vi "HFRR ADV v011 new software.vi"() -> ()   [LabVIEW 2025] (continued)
              frame #3 {
                n3057 = disable-structure shown="Disabled" {
                  frame Disabled {
                    n3058 = local read "String 10"() -> (w3814:string)
                    n3059 = Concatenate Strings("C:\\LAB-IQ-NXT\\Data\\" ("string"), w3814, ".jpg" ("string")) -> (w3812:string)
                    n3060 = String To Path(string=w3812) -> (path=w3811:path)
                    n3061 = Delete(path (use dialog)=w3811) -> ()  [unwired: 4 in, 3 out]
                  }
                  frame Enabled {
                  }
                }
                n3062 = local write "Print 2"(FALSE ("Print")) -> ()
              }
            }
          }
        }
      }
    }
    n3063 = property on="SetTemp" class="DigNum (strict)"("Disabled"=w1752) -> ()  [unwired: 2 in, 2 out]
    n3064 = Multiply(x=w1742, y=w1744) -> (x*y=w1743:dbl)
    n3065 = local read "MWSD"() -> (w1741:dbl)
    n3066 = Add(x=w1743, y=w1741) -> (x+y=→"WS1.4":dbl)
    n3067 = Wait (ms)(milliseconds to wait=u32 50) -> ()  [unwired: 1 out]
    n3068 = Wait (ms)(milliseconds to wait=u32 50) -> ()  [unwired: 1 out]
    n3069 = local read "Quit"() -> (w1740:bool)
  }
  n3070 = VISA Close(VISA resource name=w52, error in (no error)=w51) -> (error out=w49:errorcluster)
  n3071 = call <vilib>:"Clear Errors.vi"("error in (no error)"=w49) -> ()  [unwired: 5 in, 2 out]
  n3072 = VISA Close(VISA resource name=w37, error in (no error)=w36) -> ()  [unwired: 1 out]
  n3073 = while {
    tunnel: [w3975] -> w46
    shift-right: [w3968] -> _
    shift-left: 0.0 -> [w3971]
    shift-right: [w3967] -> _
    shift-left: 0.0 -> [w3970]
    shift-right: [w3966] -> _
    shift-left: 400.0 ("vc_cmd") -> [w3969]
    stop <- w3975 stop-if-true
    # "PID LOGIC"
    n3074 = local read "RUN"() -> (w3973:bool)
    n3075 = local read "Auto Start Temp"() -> (w3962:bool)
    n3076 = local read "Auto Start Test"() -> (w3972:bool)
    n3077 = local read "START TEMP"() -> (w3964:bool)
    n3078 = And(x=w3962, y=w3972) -> (x .and. y?=w3963:bool)
    n3079 = Or(x=w3973, y=w3963) -> (x .or. y?=w3974:bool)
    n3080 = And(x=w3974, y=w3964) -> (x .and. y?=w3965:bool)
    n3081 = Wait (ms)(milliseconds to wait=u32 20) -> ()  [unwired: 1 out]
    n3082 = case shown="True" w3965 {
      tunnel: [400.0 ("out_vc_cmd") w3995] -> w3966
      tunnel: [w3978 w3997] -> w3967
      tunnel: [w3978 w3996] -> w3968
      tunnel: w3971 -> [_ w3986]
      tunnel: w3970 -> [_ w3985]
      tunnel: w3969 -> [_ w3984]
      frame False {
        w3978 = 0.0 ("error_out")
      }
      frame True {
        n3083 = local read "Set Strk"() -> (w3981:dbl)
        n3084 = local read "LVDT STROKE"() -> (w3979:dbl)
        n3085 = Add(x=w3981, y="Add up Stroke") -> (x+y=w3982:dbl)
        n3086 = formula code="// Zero-Hardcode Explicit Positional-Form PID Engine\n// Inputs: target_stroke, measured_stroke, dt, prev_error, integral_accumulator_in, prev_vc_cmd\n//         kp, ki, kd, max_step_change, max_amplitude, min_amplitude, startup_cmd\n// Outputs: vc_cmd, error_out, out_error, integral_accumulator_out, out_vc_cmd\n\n// 1. Calculate Tracking Error\nfloat current_error = target_stroke - measured_stroke;\nerror_out = current_error;\n\n// 2. Compute Proportional Term\nfloat p_term = kp * current_error;\n\n// 3. Compute Derivative Term\nfloat d_term = 0.0;\nif (dt > 0.0) {\n    d_term = kd * ((current_error - prev_error) / dt);\n}\n\n// 4. Update and Accumulate Integral Term\nfloat current_integral = integral_accumulator_in + (current_error * dt);\nfloat i_term = ki * current_integral;\n\n// 5. Calculate Ideal Target Command\nfloat ideal_command = startup_cmd + p_term + i_term + d_term;\n\n// 6. Anti-Windup Protection (Back-calculation method)\nif (ideal_command > max_amplitude) {\n    float excess = ideal_command - max_amplitude;\n    if (ki > 0.0) {\n        current_integral -= excess / ki;\n    }\n    ideal_command = max_amplitude;\n} else if (ideal_command < min_amplitude) {\n    float excess = ideal_command - min_amplitude;\n    if (ki > 0.0) {\n        current_integral -= excess / ki;\n    }\n    ideal_command = min_amplitude;\n}\n\n// 7. Apply Loop Rate Limiting (Protects voice coil from large voltage steps)\nfloat raw_adjustment = ideal_command - prev_vc_cmd;\n\nif (raw_adjustment > max_step_change) {\n    raw_adjustment = max_step_change;\n} else if (raw_adjustment < -max_step_change) {\n    raw_adjustment = -max_step_change;\n}\n\nfloat next_vc_cmd = prev_vc_cmd + raw_adjustment;\n\n// Final Output Safety Safeguard Clamping\nif (next_vc_cmd > max_amplitude) {\n    next_vc_cmd = max_amplitude;\n} else if (next_vc_cmd < min_amplitude) {\n    next_vc_cmd = min_amplitude;\n}\n\n// 8. Map to Shift Registers for memory persistence\nvc_cmd = next_vc_cmd;\nout_error = current_error;                     \nintegral_accumulator_out = current_integral;  \nout_vc_cmd = next_vc_cmd;"("target_stroke"=w3982, "measured_stroke"=w3979, "dt"="dt", "integral_accumulator_in"=w3985, "prev_error"=w3986, "prev_vc_cmd"=w3984, "kp"="kp", "ki"="ki", "kd"="kd", "max_step_change"="max_step_change", "max_amplitude"="max_amplitude", "min_amplitude"="min_amplitude", "startup_cmd"="startup_cmd") -> ("vc_cmd"=w4001:dbl, "out_error"=w3996:dbl, "integral_accumulator_out"=w3997:dbl, "out_vc_cmd"=w3995:dbl)  [unwired: 1 out]
        "output Vpp" <- w4001
        n3087 = Number To Fractional String(number=w4001, precision (6)=i16 1) -> (F-format string=w3999:string)  [unwired: 2 in]
        n3088 = Concatenate Strings("DAC;" ("string"), w3999) -> (w3983:string)
        n3089 = local write "Command"(w3983) -> ()
        "prev_error" <- w3986
        "integral_accumulator_in" <- w3985
        "prev_vc_cmd" <- w3984
      }
    }
    n3090 = local read "Quit"() -> (w3975:bool)
  }
  n3091 = Or(x=w42, y=w41) -> (x .or. y?=w43:bool)
  n3092 = Or(x=w39, y=w43) -> (x .or. y?=w48:bool)
  n3093 = control-ref of="new picture"() -> ()  [unwired: 1 out]
  n3094 = Or(x=w54, y=w48) -> (x .or. y?=w45:bool)
  n3095 = Or(x=w45, y=w46) -> (x .or. y?=w40:bool)
  n3096 = while {
    tunnel: [w4002] -> w53
    i -> [w4009]
    stop <- w4002 stop-if-true
    n3097 = local read "Quit"() -> (w4002:bool)
    n3098 = Equal To 0?(x=w4009) -> (x = 0?=w4007:bool)
    n3099 = call "Elapsed Time3"("Time Target (s)"=45.0, "Auto Reset"=TRUE) -> ("Time has Elapsed"=w4006:bool)  [unwired: 10 in, 7 out]
    n3100 = Wait (ms)(milliseconds to wait=u32 50) -> ()  [unwired: 1 out]
    n3101 = Or(x=w4006, y=w4007) -> (x .or. y?=w4008:bool)
    n3102 = case shown="True" w4008 {
      frame False {
      }
      frame True {
        n3103 = call <vilib>:"System Exec.vi"("run minimized? (F)"=TRUE, "error in (no error)"="error in (no error)", "command line"="powercfg.exe -change -monitor-timeout-ac 0") -> ("error out"=w4020:errorcluster)  [unwired: 5 in, 3 out]
        n3104 = call <vilib>:"System Exec.vi"("run minimized? (F)"=TRUE, "error in (no error)"=w4020, "command line"="powercfg.exe -change -disk-timeout-ac 0") -> ("error out"=w4019:errorcluster)  [unwired: 5 in, 3 out]
        n3105 = call <vilib>:"System Exec.vi"("run minimized? (F)"=TRUE, "error in (no error)"=w4019, "command line"="powercfg.exe -change -standby-timeout-ac 0") -> ("error out"=w4018:errorcluster)  [unwired: 5 in, 3 out]
        n3106 = call <vilib>:"System Exec.vi"("run minimized? (F)"=TRUE, "error in (no error)"=w4018, "command line"="powercfg.exe -change -hibernate-timeout-ac 0") -> ("error out"=w4017:errorcluster)  [unwired: 5 in, 3 out]
        n3107 = call <vilib>:"Simple Error Handler.vi"("error in (no error)"=w4017) -> ("error out"=w4023:errorcluster)  [unwired: 4 in, 4 out]
        n3108 = call <vilib>:"Clear Errors.vi"("error in (no error)"=w4023) -> ("error out"=→"error out":errorcluster)  [unwired: 5 in, 1 out]
      }
    }
  }
  n3109 = Compound Arithmetic op=OR(w56, w40, w53) -> (w55:bool)
  n3110 = flat-sequence {
    tunnel: w55 -> [_]
    tunnel: [w4025] -> w18
    tunnel: w18 -> [_]
    frame #0 {
      n3111 = call "CLOSE CONNECTION.vi"() -> ("error out"=w4025:errorcluster)  [unwired: 11 in]
    }
    frame #1 {
      n3112 = Quit LabVIEW(quit? (T)=TRUE) -> ()
      n3113 = local write "Quit"(FALSE ("EXIT")) -> ()
    }
  }
  n3114 = property on="Heater Button" class="Bool (strict)"("Visible"=TRUE) -> ()  [unwired: 2 in, 2 out]
  n3115 = disable-structure shown="Disabled" {
    disable-tunnel: _ -> [w4031 _]
    disable-tunnel: _ -> [w4028 _]
    disable-tunnel: _ -> [w4029 _]
    frame Disabled {
      n3116 = disable-structure shown="Disabled" {
        disable-tunnel: [w4038 _] -> w4030
        frame Disabled {
          n3117 = while {
            shift-right: [w4080] -> w4036
            shift-left: errorcluster {"status"=TRUE, "code"=0, "source"="Init"} ("error out") -> [w4045]
            shift-right: [w4079] -> w4035
            shift-left: _ -> [w4046]
            shift-right: [w4078] -> _
            shift-left: "" -> [w4077]
            tunnel: [w4039] -> w4038
            shift-right: ["Set Rh"] -> _
            shift-left: 0.0 ("Set Rh") -> [w4071]
            tunnel: [w4048] -> _
            i -> [w4048]
            stop <- w4039 stop-if-true
            n3118 = flat-sequence {
              tunnel: w4045 -> [w4083]
              tunnel: [w4083] -> w4044
              frame #0 {
                n3119 = Wait (ms)(milliseconds to wait=u32 200) -> ()  [unwired: 1 out]
              }
            }
            n3120 = local read "Com Port 3"() -> (w4047:refnum<visa-resource-name>)
            n3121 = local read "Humidity Str Rec"() -> (w4049:string)
            n3122 = Not Equal?(x="Set Rh", y=w4071) -> (x != y?=w4076:bool)
            n3123 = Number To Decimal String(number="Set Rh") -> (decimal integer string=w4074:string)  [unwired: 1 in]
            n3124 = Not Equal?(x=w4047, y=w4046) -> (x != y?=w4042:bool)
            n3125 = Concatenate Strings("#setPoint00" ("string"), w4074) -> (w4075:string)
            n3126 = case shown="False" w4076 {
              tunnel: w4075 -> [_ w4095]
              frame False {
                n3127 = local read "Humidity"() -> (w4092:bool)
                n3128 = case shown="True" w4092 {
                  frame False {
                    n3129 = local write "Humidity Str Send"("stop" ("Humidity Str Send")) -> ()
                  }
                  frame True {
                    n3130 = local write "Humidity Str Send"("start" ("Humidity Str Send")) -> ()
                  }
                }
              }
              frame True {
                n3131 = local write "Humidity Str Send"(w4095) -> ()
              }
            }
            n3132 = Or(x=w4042) -> (y=w4040:bool, x .or. y?=w4041:bool)
            n3133 = String Subset(string=w4049, offset (0)=7) -> (substring=w4064:string)  [unwired: 1 in]
            n3134 = Match Pattern(string=w4049, regular expression="?") -> (offset past match=w4067:i32)  [unwired: 1 in, 3 out]
            n3135 = Match Pattern(string=w4049, regular expression="v") -> (offset past match=w4070:i32)  [unwired: 1 in, 3 out]
            n3136 = case shown="True" w4041 {
              tunnel: w4044 -> [w4081 _]
              tunnel: [w4081 errorcluster {"status"=TRUE, "code"=0, "source"="Init"} ("error out")] -> w4043
              frame False {
              }
              frame True {
              }
            }
            n3137 = Equal?(x=w4067, y=-1) -> (x = y?=w4051:bool)
            n3138 = Match Pattern(string=w4064, regular expression="g") -> (after substring=w4065:string, offset past match=w4056:i32)  [unwired: 1 in, 2 out]
            n3139 = Match Pattern(string=w4064, regular expression="y") -> (after substring=w4063:string, offset past match=w4057:i32)  [unwired: 1 in, 2 out]
            n3140 = Greater?(x=w4057, y=w4056) -> (0:w4062:bool)
            n3141 = Greater Or Equal To 0?(x=w4057) -> (x >= 0?=w4054:bool)
            n3142 = Greater Or Equal To 0?(x=w4056) -> (x >= 0?=w4055:bool)
            n3143 = Or(x=w4054, y=w4055) -> (x .or. y?=w4053:bool)
            n3144 = Greater Or Equal To 0?(x=w4070) -> (x >= 0?=w4052:bool)
            n3145 = Select(t=w4063, s=w4062, f=w4065) -> (s? t:f=w4058:string)
            n3146 = case shown="Error" w4043 {
              selector: w4043 -> [w4108 w4154]
              tunnel: [w4106 w4147] -> w4080
              tunnel: w4046 -> [w4109 w4153]
              tunnel: [w4107 w4156] -> w4079
              tunnel: w4077 -> [w4096 w4155]
              tunnel: [w4103 w4155] -> w4078
              frame No Error {
                n3147 = call "Elapsed Time7"() -> ("Time has Elapsed"=w4102:bool)  [unwired: 12 in, 7 out]
                n3148 = Not Equal?(x="Humidity Str Send", y=w4096) -> (x != y?=w4098:bool)
                n3149 = Or(x=w4098, y=w4102) -> (x .or. y?=w4101:bool)
                n3150 = Select(t="Humidity Str Send", s=w4098, f="vals" ("regular expression")) -> (s? t:f=w4097:string)
                n3151 = Or(x=w4101, y="Send") -> (x .or. y?=w4105:bool)
                n3152 = case shown="True" w4105 {
                  tunnel: [w4112 w4117] -> w4106
                  tunnel: w4109 -> [w4111 w4125]
                  tunnel: w4108 -> [w4112 w4124]
                  tunnel: [w4111 w4118] -> w4107
                  tunnel: w4097 -> [_ w4123]
                  tunnel: [w4110 w4114] -> w4103
                  tunnel: "Humidity Str Send" -> [_ w4115]
                  tunnel: w4098 -> [_ w4116]
                  tunnel: w4096 -> [w4110 w4113]
                  frame False {
                  }
                  frame True {
                    n3153 = flat-sequence {
                      tunnel: w4125 -> [w4133]
                      tunnel: w4124 -> [w4132]
                      tunnel: w4123 -> [w4129]
                      tunnel: [w4131] -> w4122
                      tunnel: [w4130] -> w4121
                      tunnel: w4122 -> [w4136]
                      tunnel: w4121 -> [w4135]
                      tunnel: [w4136] -> w4120
                      tunnel: [w4135] -> w4119
                      tunnel: w4120 -> [w4143]
                      tunnel: w4119 -> [w4142]
                      tunnel: [w4141] -> w4118
                      tunnel: [w4140] -> w4117
                      frame #0 {
                        n3154 = local write "Ser Led"(TRUE ("Boolean 4")) -> ()
                        n3155 = Concatenate Strings(w4129, "\r") -> (w4128:string)
                        n3156 = VISA Write(VISA resource name=w4133, write buffer=w4128, error in (no error)=w4132) -> (VISA resource name out=w4131:refnum<visa-resource-name>, error out=w4130:errorcluster)  [unwired: 1 out]
                      }
                      frame #1 {
                        n3157 = Wait (ms)(milliseconds to wait="wait") -> ()  [unwired: 1 out]
                      }
                      frame #2 {
                        w4138 = FALSE ("Send")
                        n3158 = property class="Instr"(reference=w4143, error in=w4142) -> (reference out=w4144:refnum<visa-resource-name>, error out=w4145:errorcluster, "Serial Settings:Number of Bytes at Serial Port"=w4137:u32)
                        n3159 = local write "Send"(w4138) -> ()
                        n3160 = local write "Ser Led"(w4138) -> ()
                        n3161 = VISA Read(VISA resource name=w4144, byte count=w4137, error in (no error)=w4145) -> (VISA resource name out=w4141:refnum<visa-resource-name>, read buffer=→"Humidity Str Rec":string, error out=w4140:errorcluster)  [unwired: 1 out]
                      }
                    }
                    n3162 = Select(t=w4115, s=w4116, f=w4113) -> (s? t:f=w4114:string)
                  }
                }
              }
              frame Error {
                w4161 = u16 0 items=["None"=0, "XON/XOFF"=1, "RTS/CTS"=2, "DTR/DSR"=4] ("flow control")
                w4157 = u16 0 items=["None", "Odd", "Even", "Mark", "Space"] ("parity")
                w4160 = u16 10 items=["1.0"=10, "1.5"=15, "2.0"=20] ("stop bits")
                n3163 = VISA Close(VISA resource name=w4153, error in (no error)=w4154) -> (error out=w4152:errorcluster)
                n3164 = local write "humid"("" ("humid")) -> ()
                n3165 = local write "Humidity Str Rec"("" ("Humidity Str Rec")) -> ()
                n3166 = call <vilib>:"Clear Errors.vi"("error in (no error)"=w4152) -> ("error out"=w4151:errorcluster)  [unwired: 5 in, 1 out]
                n3167 = local read "Com Port 3"() -> (w4150:refnum<visa-resource-name>)
                n3168 = call-poly "VISA Configure Serial Port"("VISA resource name"=w4150, "timeout (10sec)"=u32 1000, "termination char\n(0xA = '\\n' = LF)"=u8 10 ("termination char\n(0xA = '\\n' = LF)"), "Enable Termination\nChar (T)"=FALSE ("Enable Termination Char (T)"), "data bits (8)"=u16 8 ("data bits"), "parity (0:none)"=w4157, "error in (no error)"=w4151, "stop bits (10: 1 bit)"=w4160, "flow control (0:none)"=w4161) -> ("VISA resource name out"=w4156:refnum<visa-resource-name>, "baud rate (9600)"=w4148:u32, "error out"=w4147:errorcluster)  [unwired: 4 in]
              }
            }
            n3169 = Compound Arithmetic op=AND(w4052, w4051, w4053) -> (w4050:bool)
            n3170 = case shown="True" w4050 {
              tunnel: w4049 -> [_ _]
              tunnel: w4058 -> [_ w4088]
              frame False {
              }
              frame True {
                w4086 = " " ("regular expression")
                n3171 = Match Pattern(string=w4088, regular expression=" ") -> (after substring=w4090:string)  [unwired: 1 in, 3 out]
                n3172 = Match Pattern(string=w4090, regular expression=w4086) -> (before substring=→"humid":string, after substring=w4087:string)  [unwired: 1 in, 2 out]
                n3173 = Match Pattern(string=w4087, regular expression=w4086) -> (before substring=→"temp_@Rh sensor":string)  [unwired: 1 in, 3 out]
              }
            }
            n3174 = local read "Quit"() -> (w4039:bool)
          }
          n3175 = VISA Close(VISA resource name=w4035, error in (no error)=w4036) -> (error out=w4032:errorcluster)
          n3176 = call <vilib>:"Clear Errors.vi"("error in (no error)"=w4032) -> ()  [unwired: 5 in, 2 out]
        }
        frame Enabled {
        }
      }
    }
    frame Enabled {
    }
  }
  n3177 = while {
    tunnel: [w4168] -> _
    i -> [w4168]
    stop <- w4164 stop-if-true
    # "Langauage selection"
    n3178 = Equal?(x="Lan flag", y=22.0) -> ()  [unwired: 1 out]
    n3179 = disable-structure shown="Disabled" {
      frame Disabled {
        n3180 = stacked-sequence {
          frame #0 {
            n3181 = case shown="\"Russian\"" "Language Selection" {
              tunnel: [0 1] -> w4170
              frame "English", Default {
              }
              frame "Russian" {
              }
            }
            n3182 = for {
              N: 130 -> [_]
              tunnel: "Table" -> [w4179]
              tunnel: w4170 -> [w4178]
              i -> [w4177]
              n3183 = Index Array(array=w4179, index (row)=w4177, index (col)=w4178) -> (element=w4176:string)
              n3184 = case shown="123" w4177 {
                tunnel: w4176 -> [w4180 w4181 _ w4182 w4183 w4184 w4185 w4186 w4187 w4188 w4189 w4190 w4191 w4192 w4193 w4194 w4195 w4196 w4197 w4198 w4199 w4200 w4201 w4202 w4203 w4204 w4205 w4206 w4207 _ _ w4208 w4209 w4210 w4211 w4212 w4213 w4222 w4229 w4236 w4243 w4247 w4250 w4253 w4255 w4257 w4258 w4259 w4260 w4261 w4262 w4263 w4264 w4265 w4266 w4267 w4268 w4269 w4270 w4271 w4272 w4273 w4274 w4275 w4276 w4277 w4278 w4279 w4280 w4281 w4282 w4283 w4284 w4285 w4286 w4287 w4288 w4289 w4290 w4291 w4292 w4293 w4294 w4295 w4296 w4297 w4298 w4299 w4300 w4301 w4302 w4303 w4304 w4305 w4306 w4307 w4308 w4309 w4310 w4311 w4312 w4313 w4314 w4315 w4316 _ w4317 w4318 w4319 w4320 w4321 w4322 w4323 w4324 w4325 w4326 w4327 w4328 w4329 _ w4330 w4331 w4332 w4333 w4334 w4335 _]
                frame 0 {
                  n3185 = local write "S"(w4180) -> ()
                }
                frame 1 {
                  n3186 = local write "S 2"(w4181) -> ()
                }
                frame 2 {
                }
                frame 3 {
                  n3187 = local write "S 4"(w4182) -> ()
                }
                frame 4 {
                  n3188 = property on="FILE" class="Str"("Caption.Text"=w4183) -> ()  [unwired: 2 in, 2 out]
                }
                frame 5 {
                  n3189 = property on="Fuel Discription :" class="Str"("Caption.Text"=w4184) -> ()  [unwired: 2 in, 2 out]
                }
                frame 6 {
                  n3190 = property on="Remarks :" class="Str"("Caption.Text"=w4185) -> ()  [unwired: 2 in, 2 out]
                }
                frame 7 {
                  n3191 = property on="Save & Continue" class="Bool (strict)"("Boolean Text.Text"=w4186) -> ()  [unwired: 2 in, 2 out]
                }
                frame 8 {
                }
                frame 9 {
                  n3192 = property on="Set Hz" class="DigNum (strict)"("Caption.Text"=w4188) -> ()  [unwired: 2 in, 2 out]
                }
                frame 10 {
                  "String 3" <- w4189
                }
                frame 11 {
                  n3193 = property on="NORMAL LOAD" class="DigNum (strict)"("Caption.Text"=w4190) -> ()  [unwired: 2 in, 2 out]
                }
                frame 12 {
                  "String 5" <- w4191
                }
                frame 13 {
                  n3194 = property on="Set Temp" class="DigNum (strict)"("Caption.Text"=w4192) -> ()  [unwired: 2 in, 2 out]
                }
                frame 14 {
                  n3195 = local write "S 15"(w4193) -> ()
                }
                frame 15 {
                  n3196 = property on="Set Rh" class="DigNum (strict)"("Caption.Text"=w4194) -> ()  [unwired: 2 in, 2 out]
                }
                frame 16 {
                  "String 13" <- w4195
                  "String 26" <- w4195
                }
                frame 17 {
                  n3197 = local write "S 18"(w4196) -> ()
                }
                frame 18 {
                  "String 17" <- w4197
                }
                frame 19 {
                  n3198 = property on="test time" class="DigNum (strict)"("Caption.Text"=w4198) -> ()  [unwired: 2 in, 2 out]
                }
                frame 20 {
                  "String 18" <- w4199
                  "String 22" <- w4199
                }
                frame 21 {
                  n3199 = property on="Elapsed time" class="DigNum (strict)"("Caption.Text"=w4200) -> ()  [unwired: 2 in, 2 out]
                }
                frame 22 {
                  n3200 = property on="Samplingtime 2" class="DigNum (strict)"("Caption.Text"=w4201) -> ()  [unwired: 2 in, 2 out]
                }
                frame 23 {
                  "String 21" <- w4202
                }
                frame 24 {
                  n3201 = property on="Countdown" class="DigNum (strict)"("Caption.Text"=w4203) -> ()  [unwired: 2 in, 2 out]
                }
                frame 25 {
                  n3202 = property on="Countdown 2" class="DigNum (strict)"("Caption.Text"=w4204) -> ()  [unwired: 2 in, 2 out]
                }
                frame 26 {
                  n3203 = property on="Engage" class="Bool (strict)"("Boolean Text.Text"=w4205) -> ()  [unwired: 2 in, 2 out]
                }
                frame 27 {
                  n3204 = property on="Boolean  4" class="Bool (strict)"("Boolean Text.Text"=w4206) -> ()  [unwired: 2 in, 2 out]
                }
                frame 28 {
                  n3205 = property on="Test \nStatus" class="Bool (strict)"("Boolean Text.Text"=w4207) -> ()  [unwired: 2 in, 2 out]
                }
                frame 29 {
                }
                frame 30 {
                }
                frame 31 {
                }
                frame 32 {
                  n3206 = property on="RSTCOF" class="Bool"("Boolean Text.Text"=w4209) -> ()  [unwired: 2 in, 2 out]
                  n3207 = property on="RST FF" class="Bool"("Boolean Text.Text"=w4209) -> ()  [unwired: 2 in, 2 out]
                  n3208 = property on="RST TEMP" class="Bool"("Boolean Text.Text"=w4209) -> ()  [unwired: 2 in, 2 out]
                  n3209 = property on="RSTV1 3" class="Bool"("Boolean Text.Text"=w4209) -> ()  [unwired: 2 in, 2 out]
                  n3210 = property on="rstv2" class="Bool"("Boolean Text.Text"=w4209) -> ()  [unwired: 2 in, 2 out]
                  n3211 = property on="RSTV1 2" class="Bool"("Boolean Text.Text"=w4209) -> ()  [unwired: 2 in, 2 out]
                  n3212 = property on="RST CP" class="Bool"("Boolean Text.Text"=w4209) -> ()  [unwired: 2 in, 2 out]
                }
                frame 33 {
                  "S 61" <- w4210
                }
                frame 34 {
                  "String 23" <- w4211
                }
                frame 35 {
                  n3213 = property on="Rh Before" class="DigNum (strict)"("Caption.Text"=w4212) -> ()  [unwired: 2 in, 2 out]
                }
                frame 36 {
                  n3214 = Match Pattern(string=w4213, regular expression=",") -> (before substring=→"bs":string, after substring=→"as":string)  [unwired: 1 in, 2 out]
                  n3215 = property on="Rh After" class="DigNum (strict)"("Caption.Text"=w4213) -> ()  [unwired: 2 in, 2 out]
                }
                frame 37 {
                  n3216 = Match Pattern(string=w4222, regular expression=",") -> (before substring=w4221:string, after substring=w4220:string)  [unwired: 1 in, 2 out]
                  "bs" <- w4221
                  "as" <- w4220
                  n3217 = Concatenate Strings(w4221, w4220) -> (w4217:string)
                  n3218 = property on="Humidity before test 2" class="DigNum (strict)"("Caption.Text"=w4217) -> ()  [unwired: 2 in, 2 out]
                  n3219 = property on="Humidity before test" class="DigNum (strict)"("Caption.Text"=w4217) -> ()  [unwired: 2 in, 2 out]
                  n3220 = Concatenate Strings(w4217, "=" ("string")) -> (w4218:string)
                  n3221 = local write "S 38"(w4218) -> ()
                }
                frame 38 {
                  n3222 = Match Pattern(string=w4229, regular expression=",") -> (before substring=w4228:string, after substring=w4227:string)  [unwired: 1 in, 2 out]
                  "bs" <- w4228
                  "as" <- w4227
                  n3223 = Concatenate Strings(w4228, w4227) -> (w4224:string)
                  n3224 = property on="Humidity after test 2" class="DigNum (strict)"("Caption.Text"=w4224) -> ()  [unwired: 2 in, 2 out]
                  n3225 = Concatenate Strings(w4224, "=" ("string")) -> (w4226:string)
                  n3226 = property on="Humidity after test" class="DigNum (strict)"("Caption.Text"=w4224) -> ()  [unwired: 2 in, 2 out]
                  n3227 = local write "S 39"(w4226) -> ()
                }
                frame 39 {
                  n3228 = Match Pattern(string=w4236, regular expression=",") -> (before substring=w4235:string, after substring=w4234:string)  [unwired: 1 in, 2 out]
                  "bs" <- w4235
                  "as" <- w4234
                  n3229 = Concatenate Strings(w4235, w4234) -> (w4231:string)
                  n3230 = property on="Temperature before test 2" class="DigNum (strict)"("Caption.Text"=w4231) -> ()  [unwired: 2 in, 2 out]
                  n3231 = property on="Temperature before test" class="DigNum (strict)"("Caption.Text"=w4231) -> ()  [unwired: 2 in, 2 out]
                  n3232 = Concatenate Strings(w4231, "=" ("string")) -> (→"String 34":string)
                }
                frame 40 {
                  n3233 = Match Pattern(string=w4243, regular expression=",") -> (before substring=w4242:string, after substring=w4241:string)  [unwired: 1 in, 2 out]
                  "bs" <- w4242
                  "as" <- w4241
                  n3234 = Concatenate Strings(w4242, w4241) -> (w4238:string)
                  n3235 = property on="Temperature after test 2" class="DigNum (strict)"("Caption.Text"=w4238) -> ()  [unwired: 2 in, 2 out]
                  n3236 = Concatenate Strings(w4238, "=" ("string")) -> (→"String 35":string)
                  n3237 = property on="Temperature after test" class="DigNum (strict)"("Caption.Text"=w4238) -> ()  [unwired: 2 in, 2 out]
                }
                frame 41 {
                  n3238 = property on="AVP" class="DigNum (strict)"("Caption.Text"=w4247) -> ()  [unwired: 2 in, 2 out]
                  n3239 = property on="AVP 2" class="DigNum (strict)"("Caption.Text"=w4247) -> ()  [unwired: 2 in, 2 out]
                  n3240 = Concatenate Strings(w4247, "=" ("string")) -> (→"String 36":string)
                }
                frame 42 {
                  n3241 = property on="MWSD" class="DigNum (strict)"("Caption.Text"=w4250) -> ()  [unwired: 2 in, 2 out]
                  n3242 = property on="MWSD 2" class="DigNum (strict)"("Caption.Text"=w4250) -> ()  [unwired: 2 in, 2 out]
                  n3243 = Concatenate Strings(w4250, "=" ("string")) -> (→"String 37":string)
                }
                frame 43 {
                  n3244 = property on="HCF 2" class="DigNum (strict)"("Caption.Text"=w4253) -> ()  [unwired: 2 in, 2 out]
                  n3245 = property on="HCF" class="DigNum (strict)"("Caption.Text"=w4253) -> ()  [unwired: 2 in, 2 out]
                  n3246 = Concatenate Strings(w4253, "=" ("string")) -> (→"String 38":string)
                }
                frame 44 {
                  n3247 = Concatenate Strings(w4255, "=" ("string")) -> (→"String 39":string)
                  n3248 = property on="WS1.4 2" class="DigNum (strict)"("Caption.Text"=w4255) -> ()  [unwired: 2 in, 2 out]
                  n3249 = property on="WS1.4" class="DigNum (strict)"("Caption.Text"=w4255) -> ()  [unwired: 2 in, 2 out]
                }
                frame 45 {
                  n3250 = property on="Save Results" class="Bool (strict)"("Boolean Text.Text"=w4257) -> ()  [unwired: 2 in, 2 out]
                }
                frame 46 {
                  n3251 = local write "S 47"(w4258) -> ()
                }
                frame 47 {
                  n3252 = local write "S 48"(w4259) -> ()
                }
                frame 48 {
                  n3253 = local write "S 49"(w4260) -> ()
                }
                frame 49 {
                  n3254 = local write "S 50"(w4261) -> ()
                }
                frame 50 {
                  n3255 = local write "S 51"(w4262) -> ()
                }
                frame 51 {
                  n3256 = local write "S 52"(w4263) -> ()
                }
                frame 52 {
                  n3257 = local write "S 53"(w4264) -> ()
                }
                frame 53 {
                  n3258 = local write "S 54"(w4265) -> ()
                }
                frame 54 {
                  n3259 = local write "S 55"(w4266) -> ()
                }
                frame 55 {
                  n3260 = local write "S 56"(w4267) -> ()
                }
                frame 56 {
                  n3261 = local write "S 57"(w4268) -> ()
                }
                frame 57 {
                  n3262 = local write "S 58"(w4269) -> ()
                }
                frame 58 {
                  n3263 = local write "S 59"(w4270) -> ()
                }
                frame 59 {
                  n3264 = local write "S 60"(w4271) -> ()
                }
                frame 60 {
                  n3265 = local write "S 62"(w4272) -> ()
                }
                frame 61 {
                  n3266 = local write "S 63"(w4273) -> ()
                }
                frame 62 {
                  n3267 = local write "S 64"(w4274) -> ()
                }
                frame 63 {
                  n3268 = local write "S 65"(w4275) -> ()
                }
                frame 64 {
                  n3269 = local write "S 66"(w4276) -> ()
                }
                frame 65 {
                  n3270 = local write "S 67"(w4277) -> ()
                }
                frame 66 {
                  n3271 = local write "S 68"(w4278) -> ()
                }
                frame 67 {
                  n3272 = local write "S 69"(w4279) -> ()
                }
                frame 68 {
                  n3273 = local write "S 70"(w4280) -> ()
                }
                frame 69 {
                  n3274 = local write "S 71"(w4281) -> ()
                }
                frame 70 {
                  n3275 = local write "S 72"(w4282) -> ()
                }
                frame 71 {
                  n3276 = local write "S 73"(w4283) -> ()
                }
                frame 72 {
                  n3277 = local write "S 74"(w4284) -> ()
                }
                frame 73 {
                  n3278 = local write "S 75"(w4285) -> ()
                }
                frame 74 {
                  n3279 = local write "S 76"(w4286) -> ()
                }
                frame 75 {
                  n3280 = local write "S 77"(w4287) -> ()
                }
                frame 76 {
                  n3281 = local write "S 78"(w4288) -> ()
                }
                frame 77 {
                  n3282 = local write "S 79"(w4289) -> ()
                }
                frame 79 {
                  n3283 = property on="Sample Temperature ( °C )" class="XYGraph (strict)"("Y Scale.Name Label.Text"=w4290) -> ()  [unwired: 2 in, 2 out]
                }
                frame 80 {
                  n3284 = local write "S 81"(w4291) -> ()
                  n3285 = property on="Humidity ( %RH )" class="XYGraph (strict)"("Y Scale.Name Label.Text"=w4291) -> ()  [unwired: 2 in, 2 out]
                }
                frame 78 {
                  n3286 = property on="Air Temperature  ( °C )" class="XYGraph (strict)"("X Scale.Name Label.Text"=w4292) -> ()  [unwired: 2 in, 2 out]
                  n3287 = property on="Humidity ( %RH )" class="XYGraph (strict)"("X Scale.Name Label.Text"=w4292) -> ()  [unwired: 2 in, 2 out]
                  n3288 = property on="Sample Temperature ( °C )" class="XYGraph (strict)"("X Scale.Name Label.Text"=w4292) -> ()  [unwired: 2 in, 2 out]
                  n3289 = property on="Coefficient Of Friction" class="XYGraph (strict)"("X Scale.Name Label.Text"=w4292) -> ()  [unwired: 2 in, 2 out]
                }
                frame 81 {
                  n3290 = property on="Air Temperature  ( °C )" class="XYGraph (strict)"("Y Scale.Name Label.Text"=w4293) -> ()  [unwired: 2 in, 2 out]
                }
                frame 82 {
                  n3291 = local write "S 84"(w4294) -> ()
                }
                frame 83 {
                  n3292 = local write "S 85"(w4295) -> ()
                }
                frame 84 {
                  n3293 = local write "S 86"(w4296) -> ()
                }
                frame 85 {
                  n3294 = local write "S 87"(w4297) -> ()
                }
                frame 86 {
                  n3295 = local write "S 88"(w4298) -> ()
                }
                frame 87 {
                }
                frame 88 {
                  n3296 = local write "S 90"(w4300) -> ()
                }
                frame 89 {
                  n3297 = local write "S 91"(w4301) -> ()
                }
                frame 90 {
                  n3298 = local write "S 92"(w4302) -> ()
                }
                frame 91 {
                  n3299 = local write "S 93"(w4303) -> ()
                }
                frame 92 {
                  n3300 = local write "S 94"(w4304) -> ()
                }
                frame 93 {
                  n3301 = local write "S 95"(w4305) -> ()
                }
                frame 94 {
                  n3302 = local write "S 96"(w4306) -> ()
                }
                frame 95 {
                  n3303 = local write "S 97"(w4307) -> ()
                }
                frame 96 {
                  n3304 = local write "S 98"(w4308) -> ()
                }
                frame 97 {
                  n3305 = local write "S 99"(w4309) -> ()
                }
                frame 98 {
                  n3306 = local write "S 100"(w4310) -> ()
                }
                frame 99 {
                  n3307 = local write "S 101"(w4311) -> ()
                }
                frame 100 {
                  n3308 = local write "S 102"(w4312) -> ()
                }
                frame 101 {
                  n3309 = local write "S 103"(w4313) -> ()
                }
                frame 102 {
                  n3310 = local write "S 104"(w4314) -> ()
                }
                frame 103 {
                  n3311 = local write "S 105"(w4315) -> ()
                }
                frame 104 {
                  n3312 = local write "S 106"(w4316) -> ()
                }
                frame 105 {
                }
                frame 106 {
                  n3313 = property on="OK Button 17" class="Bool (strict)"("Boolean Text.Text"=w4317) -> ()  [unwired: 2 in, 2 out]
                }
                frame 107 {
                  n3314 = property on="OK Button 16" class="Bool (strict)"("Boolean Text.Text"=w4318) -> ()  [unwired: 2 in, 2 out]
                }
                frame 108 {
                  n3315 = property on="TITTLE" class="Str"("Caption.Text"=w4319) -> ()  [unwired: 2 in, 2 out]
                }
                frame 109 {
                  "String 30" <- w4320
                }
                frame 110 {
                  n3316 = property on="Test Date" class="Str"("Caption.Text"=w4321) -> ()  [unwired: 2 in, 2 out]
                  "String 31" <- w4321
                }
                frame 111 {
                  n3317 = property on="Sample ID" class="Str"("Caption.Text"=w4322) -> ()  [unwired: 2 in, 2 out]
                  "String 32" <- w4322
                }
                frame 112 {
                  n3318 = property on="Tested by" class="Str"("Caption.Text"=w4323) -> ()  [unwired: 2 in, 2 out]
                  "String 33" <- w4323
                }
                frame 113 {
                  n3319 = property on="System Configured Printers 2" class="Arr (strict)"("Caption.Text"=w4324) -> ()  [unwired: 2 in, 2 out]
                }
                frame 114 {
                  n3320 = property on="Selected Printer" class="Str"("Caption.Text"=w4325) -> ()  [unwired: 2 in, 2 out]
                }
                frame 115 {
                  n3321 = property on="Select Printer 3" class="DigNum (strict)"("Caption.Text"=w4326) -> ()  [unwired: 2 in, 2 out]
                }
                frame 116 {
                  n3322 = property on="Print" class="Bool (strict)"("Boolean Text.Text"=w4327) -> ()  [unwired: 2 in, 2 out]
                }
                frame 117 {
                  "String 41" <- w4328
                }
                frame 118 {
                  n3323 = property on="tested by" class="Str"("Caption.Text"=w4329) -> ()  [unwired: 2 in, 2 out]
                }
                frame 119 {
                }
                frame 120 {
                  n3324 = property on="Export" class="Bool (strict)"("Boolean Text.Text"=w4330) -> ()  [unwired: 2 in, 2 out]
                }
                frame 121 {
                  n3325 = property on="TEMP INTERCEPT:" class="DigNum (strict)"("Caption.Text"=w4331) -> ()  [unwired: 2 in, 2 out]
                }
                frame 122 {
                  n3326 = property on="AIR TEMP INTERCEPT:" class="DigNum (strict)"("Caption.Text"=w4332) -> ()  [unwired: 2 in, 2 out]
                }
                frame 123 {
                  n3327 = property on="Select File Type" class="Enum (strict)"("Caption.Text"=w4333) -> ()  [unwired: 2 in, 2 out]
                }
                frame 124 {
                  n3328 = property on="s.NO" class="Str"("Caption.Text"=w4334) -> ()  [unwired: 2 in, 2 out]
                  "String 45" <- w4334
                }
                frame 125 {
                  n3329 = property on="trip1 8" class="Bool (strict)"("Boolean Text.Text"=w4335) -> ()  [unwired: 2 in, 2 out]
                }
                frame 126, Default {
                }
              }
            }
          }
          frame #1 {
            w4343 = TRUE ("Visible")
            n3330 = local read "S 91"() -> (w4360:string)
            n3331 = local read "S 90"() -> (w4359:string)
            n3332 = local read "S 88"() -> (w4358:string)
            n3333 = property on="File Path" class="Path"("Caption.Text"=w4359) -> ()  [unwired: 2 in, 2 out]
            n3334 = property on="SrvM CP" class="Bool (strict)"("Boolean Text.Text"=w4358) -> ()  [unwired: 2 in, 2 out]
            n3335 = local read "S 71"() -> (w4353:string)
            n3336 = local read "S 86"() -> (w4355:string)
            n3337 = local read "S 85"() -> (w4356:string)
            n3338 = local read "S 87"() -> (w4354:string)
            n3339 = local read "S 84"() -> (w4357:string)
            n3340 = local read "S 103"() -> (w4342:string)
            n3341 = local read "S 104"() -> (w4341:string)
            n3342 = property on="ENTER THE NEW PASSWORD" class="Str"("Caption.Text"=w4354) -> ()  [unwired: 2 in, 2 out]
            n3343 = property on="Password" class="Str"("Caption.Text"=w4356) -> ()  [unwired: 2 in, 2 out]
            n3344 = property on="ENTER CURRENT PASSWORD" class="Str"("Caption.Text"=w4355) -> ()  [unwired: 2 in, 2 out]
            n3345 = property on="EDIT" class="Bool (strict)"("Boolean Text.Text"=w4353) -> ()  [unwired: 2 in, 2 out]
            n3346 = property on="SAVE" class="Bool (strict)"("Boolean Text.Text"=w4357) -> ()  [unwired: 2 in, 2 out]
            n3347 = Build Array(w4342, w4341) -> (w4340:string[])
            n3348 = property on="Heater Button" class="Bool (strict)"("Strings [4]"=w4340) -> ()  [unwired: 2 in, 2 out]
            n3349 = property on="CH-HUMIDITY WET" class="DigNum (strict)"("Caption.Size to Text?"=w4343) -> ()  [unwired: 2 in, 2 out]
            n3350 = property on="CH-HUMIDITY DRY" class="DigNum (strict)"("Caption.Size to Text?"=w4343) -> ()  [unwired: 2 in, 2 out]
            n3351 = property on="CH-POWER -" class="DigNum (strict)"("Caption.Size to Text?"=w4343) -> ()  [unwired: 2 in, 2 out]
            n3352 = property on="CH-HEATER" class="DigNum (strict)"("Caption.Size to Text?"=w4343) -> ()  [unwired: 2 in, 2 out]
            n3353 = property on="CH-POWER +" class="DigNum (strict)"("Caption.Size to Text?"=w4343) -> ()  [unwired: 2 in, 2 out]
            n3354 = local read "S 92"() -> (w4352:string)
            n3355 = local read "S 93"() -> (w4351:string)
            n3356 = local read "S 105"() -> (w4338:string)
            n3357 = local read "S 106"() -> (w4337:string)
            n3358 = Build Array(w4352, w4351) -> ()  [unwired: 1 out]
            n3359 = Build Array(w4338, w4337) -> (w4339:string[])
            n3360 = local read "S 95"() -> (w4349:string)
            n3361 = local read "S 94"() -> (w4350:string)
            n3362 = local read "bs"() -> (w4365:string)
            n3363 = local read "as"() -> (w4366:string)
            n3364 = property on="Humidity" class="Bool (strict)"("Strings [4]"=w4339) -> ()  [unwired: 2 in, 2 out]
            n3365 = Concatenate Strings(w4365, "\r", w4366) -> ()  [unwired: 1 out]
            n3366 = property on="STROKE GAIN :" class="DigNum (strict)"("Caption.Text"=w4349) -> ()  [unwired: 2 in, 2 out]
            n3367 = property on="DISPLACEMENT :" class="DigNum (strict)"("Caption.Text"=w4350) -> ()  [unwired: 2 in, 2 out]
            n3368 = property on="Rh After" class="DigNum (strict)"("Caption.Size to Text?"=TRUE ("Caption.Size to Text")) -> ()  [unwired: 2 in, 2 out]
            n3369 = local read "S 48"() -> (w4389:string)
            n3370 = local read "S 50"() -> (w4387:string)
            n3371 = local read "S 51"() -> (w4386:string)
            n3372 = local read "S 49"() -> (w4388:string)
            n3373 = local read "S 52"() -> (w4385:string)
            n3374 = local read "as"() -> (w4370:string)
            n3375 = local read "bs"() -> (w4371:string)
            n3376 = local read "S 56"() -> (w4384:string)
            n3377 = local read "S 57"() -> (w4383:string)
            n3378 = local read "S 58"() -> (w4382:string)
            n3379 = local read "S 59"() -> (w4381:string)
            n3380 = property on="OPEN" class="Bool (strict)"("Boolean Text.Text"=w4385) -> ()  [unwired: 2 in, 2 out]
            n3381 = property on="OPEN 1" class="Bool (strict)"("Boolean Text.Text"=w4389) -> ()  [unwired: 2 in, 2 out]
            n3382 = property on="OPEN 2" class="Bool (strict)"("Boolean Text.Text"=w4388) -> ()  [unwired: 2 in, 2 out]
            n3383 = property on="OPEN 3" class="Bool (strict)"("Boolean Text.Text"=w4387) -> ()  [unwired: 2 in, 2 out]
            n3384 = property on="OPEN 4" class="Bool (strict)"("Boolean Text.Text"=w4386) -> ()  [unwired: 2 in, 2 out]
            n3385 = Concatenate Strings(w4371, "\r", w4370) -> ()  [unwired: 1 out]
            n3386 = local read "S 102"() -> (w4344:string)
            n3387 = property on="КОФ1" class="DigNum (strict)"("Caption.Text"=w4384) -> ()  [unwired: 2 in, 2 out]
            n3388 = local read "S 98"() -> (w4348:string)
            n3389 = local read "S 99"() -> (w4347:string)
            n3390 = local read "S 100"() -> (w4346:string)
            n3391 = local read "S 101"() -> (w4345:string)
            n3392 = property on="КОФ2" class="DigNum (strict)"("Caption.Text"=w4383) -> ()  [unwired: 2 in, 2 out]
            n3393 = property on="КОФ3" class="DigNum (strict)"("Caption.Text"=w4382) -> ()  [unwired: 2 in, 2 out]
            n3394 = property on="КОФ4" class="DigNum (strict)"("Caption.Text"=w4381) -> ()  [unwired: 2 in, 2 out]
            n3395 = local read "bs"() -> (w4369:string)
            n3396 = local read "as"() -> (w4368:string)
            n3397 = property on="CH-POWER +" class="DigNum (strict)"("Caption.Text"=w4348) -> ()  [unwired: 2 in, 2 out]
            n3398 = property on="CH-POWER -" class="DigNum (strict)"("Caption.Text"=w4347) -> ()  [unwired: 2 in, 2 out]
            n3399 = property on="CH-HEATER" class="DigNum (strict)"("Caption.Text"=w4346) -> ()  [unwired: 2 in, 2 out]
            n3400 = property on="CH-HUMIDITY DRY" class="DigNum (strict)"("Caption.Text"=w4345) -> ()  [unwired: 2 in, 2 out]
            n3401 = property on="CH-HUMIDITY WET" class="DigNum (strict)"("Caption.Text"=w4344) -> ()  [unwired: 2 in, 2 out]
            n3402 = local read "S 60"() -> (w4380:string)
            n3403 = local read "S 54"() -> (w4390:string)
            n3404 = Concatenate Strings(w4369, "\r", w4368) -> ()  [unwired: 1 out]
            n3405 = Concatenate Strings(w4390, w4380) -> ()  [unwired: 1 out]
            n3406 = local read "S 77"() -> (→"String 43":string)
            n3407 = local read "S 76"() -> (w4363:string)
            n3408 = local read "S 78"() -> (w4362:string)
            n3409 = local read "S 71"() -> (w4374:string)
            n3410 = local read "S 66"() -> (w4379:string)
            n3411 = local read "S 67"() -> (w4378:string)
            n3412 = local read "S 68"() -> (w4377:string)
            n3413 = local read "S 69"() -> (w4376:string)
            n3414 = local read "S 70"() -> (w4375:string)
            n3415 = property on="AIR TEMP" class="DigNum (strict)"("Caption.Text"=w4362) -> ()  [unwired: 2 in, 2 out]
            n3416 = property on="Set Strk" class="DigNum (strict)"("Caption.Text"=w4363) -> ()  [unwired: 2 in, 2 out]
            n3417 = property on="FRIC. FORCE :" class="DigNum (strict)"("Caption.Text"=w4379) -> ()  [unwired: 2 in, 2 out]
            n3418 = property on="TEMPERATURE :" class="DigNum (strict)"("Caption.Text"=w4378) -> ()  [unwired: 2 in, 2 out]
            n3419 = property on="SPEED OUT:" class="DigNum (strict)"("Caption.Text"=w4377) -> ()  [unwired: 2 in, 2 out]
            n3420 = property on="AIR TEMPERATURE :" class="DigNum (strict)"("Caption.Text"=w4376) -> ()  [unwired: 2 in, 2 out]
            n3421 = property on="HUMIDITY:" class="DigNum (strict)"("Caption.Text"=w4375) -> ()  [unwired: 2 in, 2 out]
            n3422 = property on="EDIT" class="Bool (strict)"("Boolean Text.Text"=w4374) -> ()  [unwired: 2 in, 2 out]
            n3423 = local read "S 79"() -> (w4361:string)
          }
          frame #2 {
          }
        }
        n3424 = local write "Lan flag"(10.0 ("Lan flag")) -> ()
      }
      frame Enabled {
      }
    }
    n3425 = Wait (ms)(milliseconds to wait=u32 2000) -> ()  [unwired: 1 out]
    n3426 = local read "Quit"() -> (w4164:bool)
  }
  n3427 = disable-structure shown="Disabled" {
    frame Disabled {
      n3428 = while {
        tunnel: [w4392] -> _
        i -> [w4392]
        stop <- w4391 continue-if-true
        n3429 = Wait (ms)(milliseconds to wait=u32 50) -> ()  [unwired: 1 out]
        n3430 = stacked-sequence {
          frame #0 {
            # "Controls Text color"
            # "Controls BG color"
            n3431 = property on="FILE" class="Str"("Text.Text Colors:Text Color"="SC  Text") -> ()  [unwired: 2 in, 2 out]
            n3432 = property on="Fuel Discription :" class="Str"("Text.Text Colors:Text Color"="SC  Text") -> ()  [unwired: 2 in, 2 out]
            n3433 = property on="tested by" class="Str"("Text.Text Colors:Text Color"="SC  Text") -> ()  [unwired: 2 in, 2 out]
            n3434 = property on="Remarks :" class="Str"("Text.Text Colors:Text Color"="SC  Text") -> ()  [unwired: 2 in, 2 out]
            n3435 = property class="DigNum (strict)"("Numeric Text.Text Colors:BG Color"="NC BG") -> ()  [unwired: 2 in, 2 out]
            n3436 = property class="DigNum (strict)"("Numeric Text.Text Colors:BG Color"="NC BG") -> ()  [unwired: 2 in, 2 out]
            n3437 = property class="DigNum (strict)"("Numeric Text.Text Colors:BG Color"="NC BG") -> ()  [unwired: 2 in, 2 out]
            n3438 = property class="DigNum (strict)"("Numeric Text.Text Colors:BG Color"="NC BG") -> ()  [unwired: 2 in, 2 out]
            n3439 = property class="DigNum (strict)"("Numeric Text.Text Colors:BG Color"="NC BG") -> ()  [unwired: 2 in, 2 out]
            n3440 = property class="DigNum (strict)"("Numeric Text.Text Colors:BG Color"="NC BG") -> ()  [unwired: 2 in, 2 out]
            n3441 = property class="DigNum (strict)"("Numeric Text.Text Colors:BG Color"="NC BG") -> ()  [unwired: 2 in, 2 out]
            n3442 = property class="DigNum (strict)"("Numeric Text.Text Colors:BG Color"="NC BG") -> ()  [unwired: 2 in, 2 out]
            n3443 = property class="DigNum (strict)"("Numeric Text.Text Colors:BG Color"="NC BG") -> ()  [unwired: 2 in, 2 out]
            n3444 = property class="DigNum (strict)"("Numeric Text.Text Colors:BG Color"="NC BG") -> ()  [unwired: 2 in, 2 out]
            n3445 = property class="DigNum (strict)"("Numeric Text.Text Colors:BG Color"="NC BG") -> ()  [unwired: 2 in, 2 out]
            n3446 = property class="DigNum (strict)"("Numeric Text.Text Colors:BG Color"="NC BG") -> ()  [unwired: 2 in, 2 out]
            n3447 = property on="FILE" class="Str"("Text.Text Colors:BG Color"="SC BG 3") -> ()  [unwired: 2 in, 2 out]
            n3448 = property on="Fuel Discription :" class="Str"("Text.Text Colors:BG Color"="SC BG 3") -> ()  [unwired: 2 in, 2 out]
            n3449 = property on="tested by" class="Str"("Text.Text Colors:BG Color"="SC BG 3") -> ()  [unwired: 2 in, 2 out]
            n3450 = property on="Remarks :" class="Str"("Text.Text Colors:BG Color"="SC BG 3") -> ()  [unwired: 2 in, 2 out]
            n3451 = property class="DigNum (strict)"("Numeric Text.Text Colors:Text Color"="NC Text") -> ()  [unwired: 2 in, 2 out]
            n3452 = property class="DigNum (strict)"("Numeric Text.Text Colors:Text Color"="NC Text") -> ()  [unwired: 2 in, 2 out]
            n3453 = property class="DigNum (strict)"("Numeric Text.Text Colors:Text Color"="NC Text") -> ()  [unwired: 2 in, 2 out]
            n3454 = property class="DigNum (strict)"("Numeric Text.Text Colors:Text Color"="NC Text") -> ()  [unwired: 2 in, 2 out]
            n3455 = property class="DigNum (strict)"("Numeric Text.Text Colors:Text Color"="NC Text") -> ()  [unwired: 2 in, 2 out]
            n3456 = property class="DigNum (strict)"("Numeric Text.Text Colors:Text Color"="NC Text") -> ()  [unwired: 2 in, 2 out]
            n3457 = property class="DigNum (strict)"("Numeric Text.Text Colors:Text Color"="NC Text") -> ()  [unwired: 2 in, 2 out]
            n3458 = property class="DigNum (strict)"("Numeric Text.Text Colors:Text Color"="NC Text") -> ()  [unwired: 2 in, 2 out]
            n3459 = property class="DigNum (strict)"("Numeric Text.Text Colors:Text Color"="NC Text") -> ()  [unwired: 2 in, 2 out]
            n3460 = property class="DigNum (strict)"("Numeric Text.Text Colors:Text Color"="NC Text") -> ()  [unwired: 2 in, 2 out]
            n3461 = property class="DigNum (strict)"("Numeric Text.Text Colors:Text Color"="NC Text") -> ()  [unwired: 2 in, 2 out]
            n3462 = property class="DigNum (strict)"("Numeric Text.Text Colors:Text Color"="NC Text") -> ()  [unwired: 2 in, 2 out]
            n3463 = property class="DigNum (strict)"("Numeric Text.Text Colors:Text Color"="NI Text  2") -> ()  [unwired: 2 in, 2 out]
            n3464 = property class="DigNum (strict)"("Numeric Text.Text Colors:Text Color"="NI Text  2") -> ()  [unwired: 2 in, 2 out]
            n3465 = property class="DigNum (strict)"("Numeric Text.Text Colors:Text Color"="NI Text  2") -> ()  [unwired: 2 in, 2 out]
            n3466 = property class="DigNum (strict)"("Numeric Text.Text Colors:Text Color"="NI Text  2") -> ()  [unwired: 2 in, 2 out]
            n3467 = property class="DigNum (strict)"("Numeric Text.Text Colors:Text Color"="NI Text  2") -> ()  [unwired: 2 in, 2 out]
            n3468 = property class="DigNum (strict)"("Numeric Text.Text Colors:Text Color"="NI Text  2") -> ()  [unwired: 2 in, 2 out]
            n3469 = property class="DigNum (strict)"("Numeric Text.Text Colors:Text Color"="NI Text  2") -> ()  [unwired: 2 in, 2 out]
            n3470 = property class="DigNum (strict)"("Numeric Text.Text Colors:Text Color"="NI Text  2") -> ()  [unwired: 2 in, 2 out]
            n3471 = property class="DigNum (strict)"("Numeric Text.Text Colors:Text Color"="NI Text  2") -> ()  [unwired: 2 in, 2 out]
            n3472 = property class="DigNum (strict)"("Numeric Text.Text Colors:Text Color"="NI Text  2") -> ()  [unwired: 2 in, 2 out]
            n3473 = property class="DigNum (strict)"("Numeric Text.Text Colors:Text Color"="NI Text  2") -> ()  [unwired: 2 in, 2 out]
            n3474 = property class="DigNum (strict)"("Numeric Text.Text Colors:Text Color"="NI Text  2") -> ()  [unwired: 2 in, 2 out]
            n3475 = property class="DigNum (strict)"("Numeric Text.Text Colors:Text Color"="NI Text  2") -> ()  [unwired: 2 in, 2 out]
            n3476 = property class="DigNum (strict)"("Numeric Text.Text Colors:Text Color"="NI Text  2") -> ()  [unwired: 2 in, 2 out]
            n3477 = property class="DigNum (strict)"("Numeric Text.Text Colors:Text Color"="NI Text  2") -> ()  [unwired: 2 in, 2 out]
            n3478 = property on="Coefficient Of Friction" class="XYGraph (strict)"("Plot Area:Colors:FG Color"="GFG  2", "Plot Area:Colors:BG Color"="GBG   2") -> ()  [unwired: 2 in, 2 out]
            n3479 = property on="Humidity ( %RH )" class="XYGraph (strict)"("Plot Area:Colors:FG Color"="GFG  2", "Plot Area:Colors:BG Color"="GBG   2") -> ()  [unwired: 2 in, 2 out]
            n3480 = property on="Air Temperature  ( °C )" class="XYGraph (strict)"("Plot Area:Colors:FG Color"="GFG  2", "Plot Area:Colors:BG Color"="GBG   2") -> ()  [unwired: 2 in, 2 out]
            n3481 = property on="Sample Temperature ( °C )" class="XYGraph (strict)"("Plot Area:Colors:FG Color"="GFG  2", "Plot Area:Colors:BG Color"="GBG   2") -> ()  [unwired: 2 in, 2 out]
            n3482 = property class="DigNum (strict)"("Numeric Text.Text Colors:BG Color"="NI BG 2") -> ()  [unwired: 2 in, 2 out]
            n3483 = property class="DigNum (strict)"("Numeric Text.Text Colors:BG Color"="NI BG 2") -> ()  [unwired: 2 in, 2 out]
            n3484 = property class="DigNum (strict)"("Numeric Text.Text Colors:BG Color"="NI BG 2") -> ()  [unwired: 2 in, 2 out]
            n3485 = property class="DigNum (strict)"("Numeric Text.Text Colors:BG Color"="NI BG 2") -> ()  [unwired: 2 in, 2 out]
            n3486 = property class="DigNum (strict)"("Numeric Text.Text Colors:BG Color"="NI BG 2") -> ()  [unwired: 2 in, 2 out]
            n3487 = property class="DigNum (strict)"("Numeric Text.Text Colors:BG Color"="NI BG 2") -> ()  [unwired: 2 in, 2 out]
            n3488 = property class="DigNum (strict)"("Numeric Text.Text Colors:BG Color"="NI BG 2") -> ()  [unwired: 2 in, 2 out]
            n3489 = property class="DigNum (strict)"("Numeric Text.Text Colors:BG Color"="NI BG 2") -> ()  [unwired: 2 in, 2 out]
            n3490 = property class="DigNum (strict)"("Numeric Text.Text Colors:BG Color"="NI BG 2") -> ()  [unwired: 2 in, 2 out]
            n3491 = property class="DigNum (strict)"("Numeric Text.Text Colors:BG Color"="NI BG 2") -> ()  [unwired: 2 in, 2 out]
            n3492 = property class="DigNum (strict)"("Numeric Text.Text Colors:BG Color"="NI BG 2") -> ()  [unwired: 2 in, 2 out]
            n3493 = property class="DigNum (strict)"("Numeric Text.Text Colors:BG Color"="NI BG 2") -> ()  [unwired: 2 in, 2 out]
            n3494 = property class="DigNum (strict)"("Numeric Text.Text Colors:BG Color"="NI BG 2") -> ()  [unwired: 2 in, 2 out]
            n3495 = property class="DigNum (strict)"("Numeric Text.Text Colors:BG Color"="NI BG 2") -> ()  [unwired: 2 in, 2 out]
            n3496 = property class="DigNum (strict)"("Numeric Text.Text Colors:BG Color"="NI BG 2") -> ()  [unwired: 2 in, 2 out]
            n3497 = property class="Bool"("Colors [4]"="Boolean BC T & BG") -> ()  [unwired: 2 in, 2 out]
            n3498 = property on="Save & Continue" class="Bool (strict)"("Colors [4]"="Boolean BC T & BG") -> ()  [unwired: 2 in, 2 out]
            n3499 = property on="Heater Button" class="Bool (strict)"("Colors [4]"="Boolean BC T & BG") -> ()  [unwired: 2 in, 2 out]
            n3500 = property class="Bool"("Colors [4]"="Boolean BC T & BG") -> ()  [unwired: 2 in, 2 out]
            n3501 = property on="Humidity" class="Bool (strict)"("Colors [4]"="Boolean BC T & BG") -> ()  [unwired: 2 in, 2 out]
            n3502 = property class="Bool (strict)"("Colors [4]"="Boolean BC T & BG") -> ()  [unwired: 2 in, 2 out]
            n3503 = property on="RUN" class="Bool (strict)"("Colors [4]"="Boolean BC T & BG") -> ()  [unwired: 2 in, 2 out]
            n3504 = property on="trip1 8" class="Bool (strict)"("Colors [4]"="Boolean BC T & BG") -> ()  [unwired: 2 in, 2 out]
            n3505 = property class="Bool"("Colors [4]"="Boolean BC T & BG") -> ()  [unwired: 2 in, 2 out]
            n3506 = property class="Bool (strict)"("Colors [4]"="Boolean BC T & BG") -> ()  [unwired: 2 in, 2 out]
            n3507 = property on="OPEN 1" class="Bool (strict)"("Colors [4]"="Boolean BC T & BG 2") -> ()  [unwired: 2 in, 2 out]
            n3508 = property on="OPEN 2" class="Bool (strict)"("Colors [4]"="Boolean BC T & BG 2") -> ()  [unwired: 2 in, 2 out]
            n3509 = property on="OPEN 3" class="Bool (strict)"("Colors [4]"="Boolean BC T & BG 2") -> ()  [unwired: 2 in, 2 out]
            n3510 = property on="OPEN 4" class="Bool (strict)"("Colors [4]"="Boolean BC T & BG 2") -> ()  [unwired: 2 in, 2 out]
            n3511 = property on="OPEN" class="Bool (strict)"("Colors [4]"="Boolean BC T & BG 2") -> ()  [unwired: 2 in, 2 out]
            n3512 = property on="rstv2" class="Bool"("Colors [4]"="Boolean BC T & BG 2") -> ()  [unwired: 2 in, 2 out]
            n3513 = property on="RST CP" class="Bool"("Colors [4]"="Boolean BC T & BG 2") -> ()  [unwired: 2 in, 2 out]
            n3514 = property on="RSTV1 3" class="Bool"("Colors [4]"="Boolean BC T & BG 2") -> ()  [unwired: 2 in, 2 out]
            n3515 = property on="RSTV1 2" class="Bool"("Colors [4]"="Boolean BC T & BG 2") -> ()  [unwired: 2 in, 2 out]
          }
          frame #1 {
          }
        }
        n3516 = local read "Quit"() -> (w4391:bool)
      }
    }
    frame Enabled {
    }
  }
  n3517 = while {
    shift-right: [w4409] -> _
    shift-left: _ -> [w4410]
    shift-right: [w4407] -> _
    shift-left: T18 {"Read Heave and Surge"="", "Bytes at Heave Port"=0.0, "Heave and Surge COM Port:"="COM9", "Com Port 2"="COM7", "Residual Due"="", "Heave COM Status 2"=TRUE, "Heave COM Status"=TRUE, "Port 2"=TRUE, "Sway PPR"=6400.0, "Surge PPR"=6400.0, "Heave PPR"=6400.0, "Sway Pitch"=2.0, "Surge Pitch"=3.0, "Heave Pitch"=4.0, "Sway Pulses/mm"=320.0, "Surge Pulses/mm"=1600.0, "Heave Pulses/mm"=1600.0, "inner loop"=0.0, "Read Heave and Surge 2"="", "String 36"="", "Write S"=FALSE, "WriteCC1"=[""], "Heave COM Loop"=0, "LastCom"="", "EXIT"=FALSE, "Error Heave"={"status"=TRUE, "code"=-1073807343, "source"=""}} -> [w4406]
    shift-right: [w4404] -> _
    shift-left: enum16{"init", "MAIN", "Panel Close"}."init" -> [w4405]
    stop <- w4408 stop-if-true
    n3518 = case shown="\"MAIN\"" w4405 {
      tunnel: w4410 -> [w4424 w4439 w4500 w4502]
      tunnel: [w4418 w4448 w4500 w4502] -> w4409
      tunnel: [_ _ TRUE _] -> w4408
      tunnel: [w4414 w4445 w4498 w4501] -> w4407
      tunnel: w4406 -> [w4421 w4438 w4498 w4501]
      tunnel: [enum16{"init", "MAIN", "Panel Close"}."MAIN" w4432 _ _] -> w4404
      frame "init" {
        n3519 = Bundle By Name(cluster=w4421, "Heave and Surge COM Port:"="C3 :") -> (w4420:T18)
        n3520 = call "Instrument fgv.vi"("Enum"=T30."INIT", "error in (no error) 2"=w4424, "INPUT"=w4420) -> ("error"=w4422:errorcluster, "output"=w4417:T18)  [unwired: 6 in, 1 out]
        n3521 = case shown="No Error" w4422 {
          selector: w4422 -> [w4426 _]
          tunnel: [w4426 w4430] -> w4418
          tunnel: w4417 -> [w4425 w4428]
          tunnel: [w4425 w4427] -> w4415
          frame No Error {
          }
          frame Error {
            n3522 = call "Instrument fgv.vi"("Enum"=T30."ERROR INIT", "INPUT"=w4428) -> ("error"=w4431:errorcluster, "output"=w4427:T18)  [unwired: 7 in, 1 out]
            n3523 = call <vilib>:"Clear Errors.vi"("error in (no error)"=w4431) -> ("error out"=w4430:errorcluster)  [unwired: 5 in, 1 out]
          }
        }
        n3524 = local read "LastCom"() -> (w4413:string)
